vi "ShamsiToMiladi.vi"(1 "Jalali(Shamsi) Date":string) -> (0 "Gregorian(Miladi) Date":string)   [LabVIEW 2015]
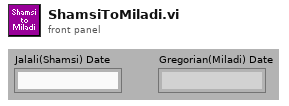
[diagram p1: front panel]
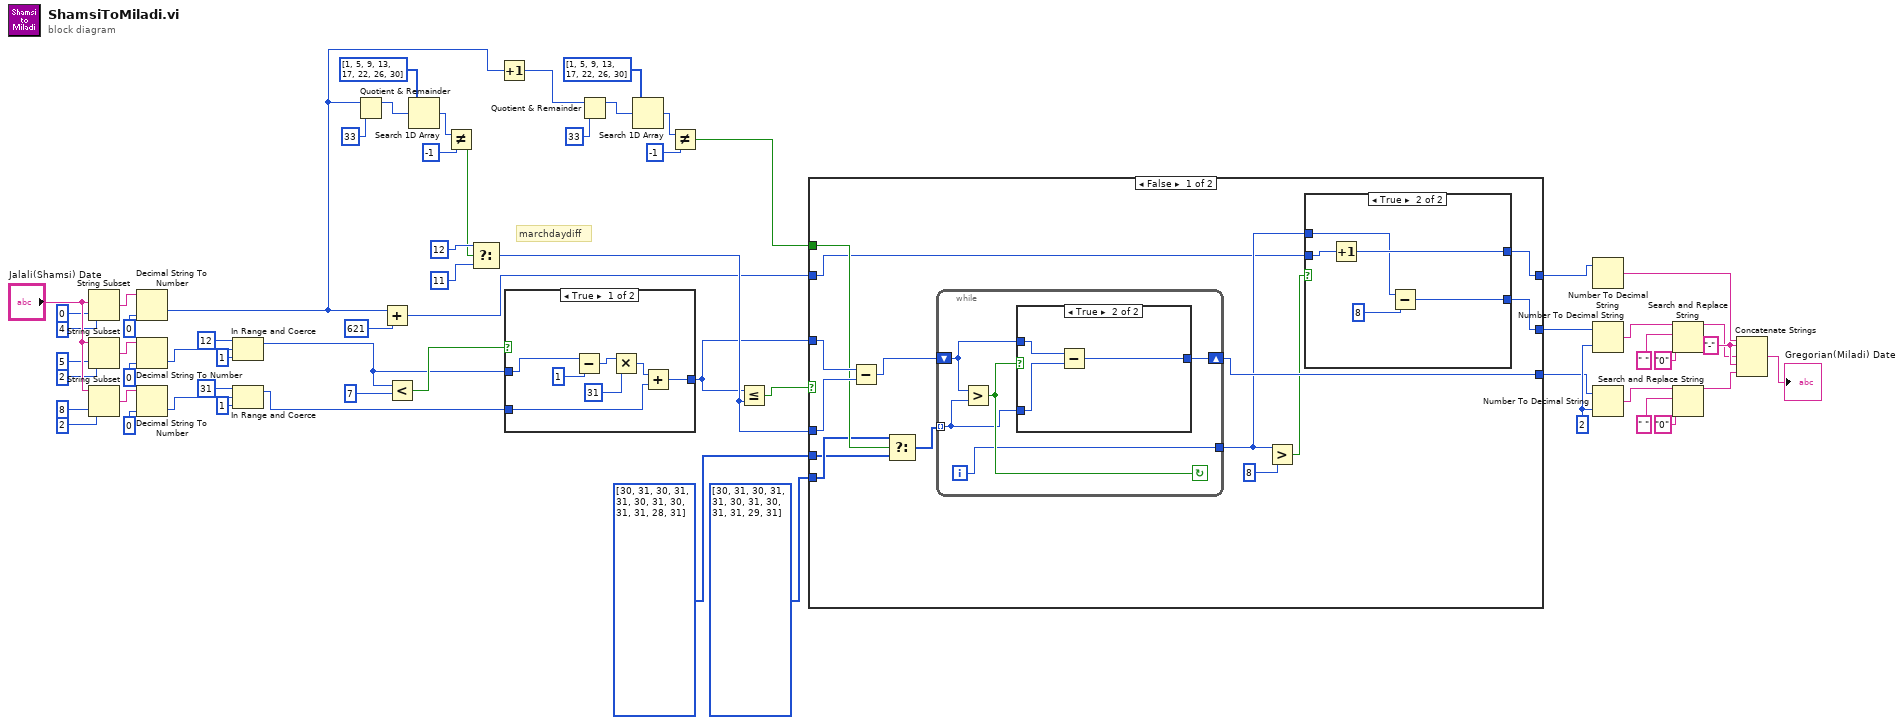
[diagram p0: block diagram]
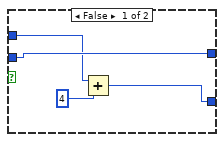
[diagram p2: hidden frame]
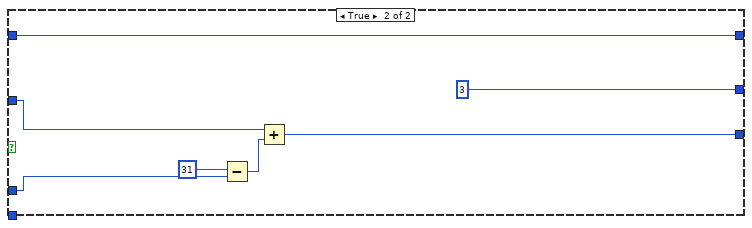
[diagram p4: hidden frame]
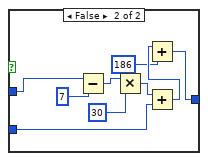
[diagram p5: hidden frame]
diagram:
  w41 = "-" ("string")
  w48 = u8 2 ("width (-)")
  # "marchdaydiff"
  n1 = String Subset(string="Jalali(Shamsi) Date", offset (0)=0, length (rest)=4 ("length (rest)")) -> (substring=w54:string)
  n2 = String Subset(string="Jalali(Shamsi) Date", offset (0)=5, length (rest)=2 ("length (rest)")) -> (substring=w53:string)
  n3 = String Subset(string="Jalali(Shamsi) Date", offset (0)=8, length (rest)=2 ("length (rest)")) -> (substring=w52:string)
  n4 = Decimal String To Number(string=w54, default (0L)=u16 0) -> (number=w22:u16)  [unwired: 1 in, 1 out]
  n5 = Decimal String To Number(string=w53, default (0L)=u16 0) -> (number=w8:u16)  [unwired: 1 in, 1 out]
  n6 = Decimal String To Number(string=w52, default (0L)=u16 0) -> (number=w2:u16)  [unwired: 1 in, 1 out]
  n7 = In Range and Coerce(upper limit=u16 12, x=w8, lower limit=u16 1) -> (coerced(x)=w5:u16)  [unwired: 1 out]
  n8 = In Range and Coerce(upper limit=u16 31, x=w2, lower limit=u16 1) -> (coerced(x)=w1:u16)  [unwired: 1 out]
  n9 = Quotient & Remainder(x=w22, y=u16 33) -> (x-y*floor(x/y)=w20:u16)  [unwired: 1 out]
  n10 = Add(x=w22, y=u16 621) -> (x+y=w23:u16)
  n11 = Less?(x=w5, y=u16 7) -> (x < y?=w32:bool)
  n12 = Search 1D Array(1D array=u16[] [1, 5, 9, 13, 17, 22, 26, 30], element=w20) -> (index of element=w18:i32)  [unwired: 1 in]
  n13 = Not Equal?(x=w18, y=-1) -> (x != y?=w16:bool)
  n14 = Select(t=u16 12 ("y"), s=w16, f=u16 11 ("y")) -> (s? t:f=w29:u16)
  n15 = Increment(x=w22) -> (x+1=w10:u16)
  n16 = case shown="True" w32 {
    tunnel: w5 -> [w68 w77]
    tunnel: w1 -> [w63 w72]
    tunnel: [w62 w70] -> w28
    frame True {
      n17 = Subtract(x=w68, y=u16 1) -> (x-y=w66:u16)
      n18 = Multiply(x=w66, y=u16 31) -> (x*y=w64:u16)
      n19 = Add(x=w64, y=w63) -> (x+y=w62:u16)
    }
    frame False {
      n20 = Subtract(x=w77, y=u16 7) -> (x-y=w75:u16)
      n21 = Multiply(x=w75, y=u16 30) -> (x*y=w73:u16)
      n22 = Add(x=w73, y=w72) -> (x+y=w71:u16)
      n23 = Add(x=w71, y=u16 186) -> (x+y=w70:u16)
    }
  }
  n24 = Quotient & Remainder(x=w10, y=u16 33) -> (x-y*floor(x/y)=w14:u16)  [unwired: 1 out]
  n25 = Search 1D Array(1D array=u16[] [1, 5, 9, 13, 17, 22, 26, 30], element=w14) -> (index of element=w12:i32)  [unwired: 1 in]
  n26 = Not Equal?(x=w12, y=-1) -> (x != y?=w9:bool)
  n27 = Less Or Equal?(x=w28, y=w29) -> (x <= y?=w24:bool)
  n28 = case shown="False" w24 {
    tunnel: [w78 u8 3] -> w31
    tunnel: w23 -> [w80 w115]
    tunnel: [w79 w115] -> w30
    tunnel: w29 -> [w90 w114]
    tunnel: w28 -> [w91 w111]
    tunnel: [w84 w110] -> w27
    tunnel: w9 -> [w88 _]
    tunnel: u16[] [30, 31, 30, 31, 31, 30, 31, 30, 31, 31, 28, 31] -> [w86 _]
    tunnel: u16[] [30, 31, 30, 31, 31, 30, 31, 30, 31, 31, 29, 31] -> [w87 _]
    frame False {
      n29 = Subtract(x=w91, y=w90) -> (x-y=w89:u16)
      n30 = Select(t=w87, s=w88, f=w86) -> (s? t:f=w85:u16[])
      n31 = while {
        shift-right: [w102] -> w84
        shift-left: w89 -> [w104]
        tunnel: w85 -> [w103] mode=indexing
        tunnel: [w101] -> w81
        i -> [w101]
        stop <- w105 continue-if-true
        n32 = Greater?(x=w104, y=w103) -> (0:w105:bool)
        n33 = case shown="True" w105 {
          tunnel: w104 -> [w106 w109]
          tunnel: w103 -> [_ w108]
          tunnel: [w106 w107] -> w102
          frame False {
          }
          frame True {
            n34 = Subtract(x=w109, y=w108) -> (x-y=w107:u16)
          }
        }
      }
      n35 = Greater?(x=w81, y=8) -> (0:w82:bool)
      n36 = case shown="True" w82 {
        tunnel: w81 -> [w94 w98]
        tunnel: w80 -> [w95 w100]
        tunnel: [w95 w99] -> w79
        tunnel: [w92 w96] -> w78
        frame False {
          n37 = Add(x=w94, y=4) -> (x+y=w92:i32)
        }
        frame True {
          n38 = Increment(x=w100) -> (x+1=w99:u16)
          n39 = Subtract(x=w98, y=8) -> (x-y=w96:i32)
        }
      }
    }
    frame True {
      n40 = Subtract(x=u16 31, y=w114) -> (x-y=w112:u16)
      n41 = Add(x=w111, y=w112) -> (x+y=w110:u16)
    }
  }
  n42 = Number To Decimal String(number=w30) -> (decimal integer string=w40:string)  [unwired: 1 in]
  n43 = Number To Decimal String(number=w31, width (-)=w48) -> (decimal integer string=w43:string)
  n44 = Number To Decimal String(number=w27, width (-)=w48) -> (decimal integer string=w42:string)
  n45 = Search and Replace String(input string=w43, search string=" ", replace string="0" ("replace string (\"\")")) -> (result string=w39:string)  [unwired: 5 in, 3 out]
  n46 = Search and Replace String(input string=w42, search string=" ", replace string="0" ("replace string (\"\")")) -> (result string=w38:string)  [unwired: 5 in, 3 out]
  n47 = Concatenate Strings(w40, w41, w39, w41, w38) -> (→"Gregorian(Miladi) Date":string)
